vi "Database.Handler.CheckStatus.vi"(8 "error in (no error)":errorcluster, 11 "Data in":T1) -> (0 "error out":errorcluster, 3 "Data out":T1)   [LabVIEW 2016]
uses:
  Database.Global.vi
  Global/ApplicationGlobal.vi
  Tools/EventLog/EventLog.EventSource.ctl
  Tools/Translator/Translator.Message.ctl
  Tools/EventLog/EventLog.New(array).vi
  Database.Handler.Data.Status.ctl
  Database.Handler.Data.Sets.ctl
  Database.Handler.Data.ctl
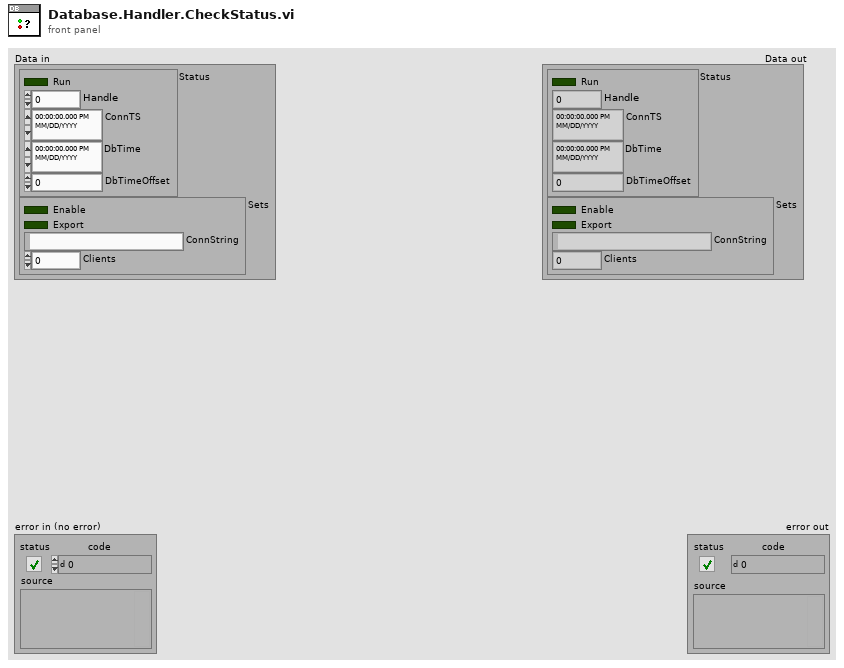
[diagram p1: front panel]
types:
  T1 = typedef "Database.Handler.Data.ctl" = cluster{"Status":T2, "Sets":T3}
  T2 = typedef "Database.Handler.Data.Status.ctl" = cluster{"Run":bool, "Handle":i32, "ConnTS":timestamp, "DbTime":timestamp, "DbTimeOffset":dbl}
  T3 = typedef "Database.Handler.Data.Sets.ctl" = cluster{"Enable":bool, "Export":bool, "ConnString":string, "Clients":i32}
  T4 = typedef "Translator.Message.ctl" = enum16{"-", "Event confirmed", "Log out", "Log in", "Shutdown", "Cancel", "Start", "Continue", "Stop", "On", "Off", "OK", "NOK", "NOK %s", "This", "Prev", "Home", "Work", "In progress...", "Missing", "Empty", "Hardware failure", "Initial", "Error %d >> %s", "Error %d >> %s >> %s", "Starting %s", "Quitting %s", "Configured", "Initializing", "Quitting", "Loading", "Running %s", "Stopped", "Summary", "Do you want to continue?", "Do you want to exit?", "Log out?", "System", "All", "IDLE", "Translating...%s", "Not found", "Alarm %s", "Run", "Skip", "Abort", "Repeat", "Please wait...", "Database disconnected", "Login to database successful", "Login to database failed: %d; %s", "Get process step data for %s", "Changeover off", "Changeover into %s", "Product %s | %s found in cache with status %d at previous station", "Product %s | %s found in database with status %d at previous station", "Product %s | %s not found in cache at previous station", "Product %s | %s not found in database at previous station", "Product %s | %s found in cache with status %d at this station (%d repetion)", "Product %s | %s found in database with status %d at this station (%d repetition)", "Product %s | %s not found in cache at this station", "Product %s | %s not found in database at this station", "Product %s | %s found in cache for component %s | %s", "Product %s | %s found in database for component %s | %s", "Product not found in cache for component %s | %s", "Product not found in database for component %s | %s", "Product %s | %s connected with component %s | %s (cache)", "Product %s | %s connected with component %s | %s (database)", "New data for %s | %s (cache)", "New data for %s | %s (database)", "File %s moved (cache)", "File %s deleted (cache)", "Msg %d >> %s", "PLC LifeBit Failure", "Reconnecting DB", "Reconnecting PLC", "Free disk space is below 1GB - contact technician"}
  T5 = typedef "EventLog.EventSource.ctl" = enum16{"All", "Gui", "Cache", "PLC1", "PLC2", "PLC3", "DB", "DB01", "DB02", "DB03", "DB04", "DB05", "DB06", "DB07", "DB08", "DB09", "DB10", "DB11", "DB12", "DB13", "DB14", "DB15", "DB16"}
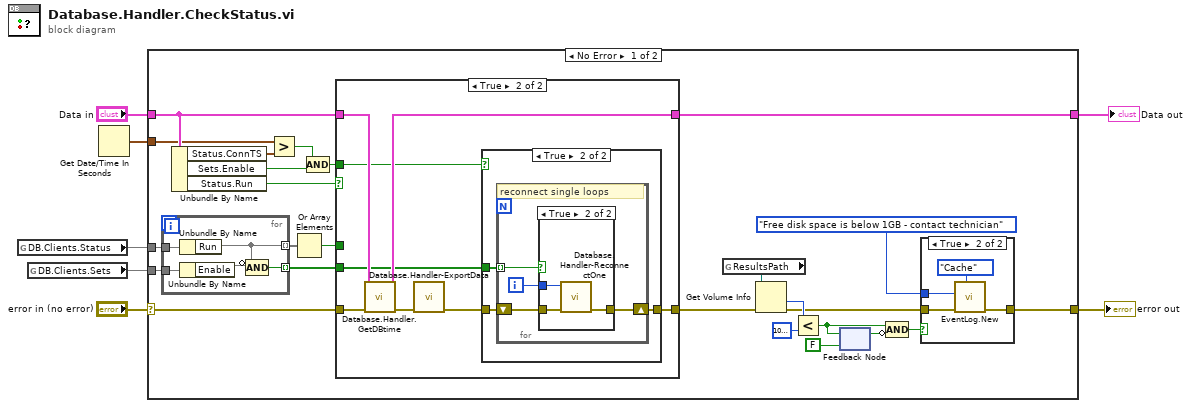
[diagram p0: block diagram]
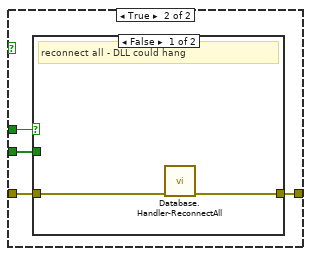
[diagram p4: hidden frame]
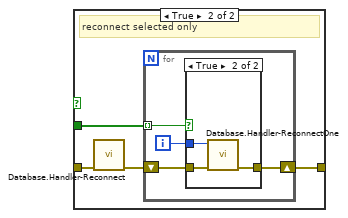
[diagram p5: hidden frame]
diagram:
  n1 = global read "Database.Global.vi" "DB.Clients.Status"() -> (w6)
  n2 = global read "Database.Global.vi" "DB.Clients.Sets"() -> (w5)
  n3 = Get Date/Time In Seconds() -> (seconds since 1Jan1904=w1:timestamp)
  n4 = case shown="No Error" "error in (no error)" {
    selector: "error in (no error)" -> [w29 w89]
    tunnel: "Data in" -> [w28 w88]
    tunnel: w6 -> [w32 _]
    tunnel: w5 -> [w31 _]
    tunnel: [w10 w89] -> w3
    tunnel: [w24 w88] -> w2
    tunnel: w1 -> [w22 _]
    frame No Error {
      n5 = for {
        tunnel: w32 -> [w42]
        tunnel: w31 -> [w41]
        tunnel: [w40] -> w30 mode=indexing
        tunnel: [w38] -> w25 mode=indexing
        n6 = Unbundle By Name(w42) -> ("Run"=w40)
        n7 = Unbundle By Name(w41) -> ("Enable"=w39)
        n8 = Compound Arithmetic op=AND(invert w40, w39) -> (w38:bool)
      }
      n9 = Unbundle By Name(w28) -> ("Status.ConnTS"=w23:timestamp, "Sets.Enable"=w21:bool, "Status.Run"=w27:bool)
      n10 = Greater?(x=w22, y=w23) -> (0:w20:bool)
      n11 = Or Array Elements(Boolean array=w30) -> (logical OR=w26:bool)
      n12 = Compound Arithmetic op=AND(w20, w21) -> (w19:bool)
      n13 = case shown="True" w27 {
        tunnel: w29 -> [w48 w74]
        tunnel: [w47 w70] -> w11
        tunnel: w28 -> [w44 w73]
        tunnel: w26 -> [w46 _]
        tunnel: w25 -> [w45 w69]
        tunnel: [w44 w72] -> w24
        tunnel: w19 -> [w43 w68]
        frame False {
          n14 = case shown="False" w43 {
            tunnel: w48 -> [w49 w52]
            tunnel: [w49 w51] -> w47
            tunnel: w46 -> [_ w53]
            tunnel: w45 -> [_ w50]
            frame False {
            }
            frame True {
              n15 = case shown="False" w53 {
                tunnel: w52 -> [w55 w57]
                tunnel: [w54 w59] -> w51
                tunnel: w50 -> [_ w58]
                frame False {
                  # "reconnect all - DLL could hang"
                  n16 = call "Database.Handler-ReconnectAll.vi"("error in"=w55) -> ("error out"=w54:errorcluster)  [unwired: 10 in]
                }
                frame True {
                  # "reconnect selected only"
                  n17 = call "Database.Handler-Reconnect.vi"("error in"=w57) -> ("error out"=w56:errorcluster)  [unwired: 10 in]
                  n18 = for {
                    shift-right: [w60] -> w59
                    shift-left: w56 -> [w63]
                    tunnel: w58 -> [w61] mode=indexing
                    i -> [w62]
                    n19 = case shown="True" w61 {
                      tunnel: w63 -> [w64 w67]
                      tunnel: w62 -> [_ w65]
                      tunnel: [w64 w66] -> w60
                      frame False {
                      }
                      frame True {
                        n20 = call "Database.Handler-ReconnectOne.vi"("error in"=w67, "ClientIdx"=w65) -> ("error out"=w66:errorcluster)  [unwired: 9 in]
                      }
                    }
                  }
                }
              }
            }
          }
        }
        frame True {
          n21 = call "Database.Handler.GetDBtime.vi"("error in (no error)"=w74, "Data in"=w73) -> ("error out"=w75:errorcluster, "Data out"=w72:T1)  [unwired: 8 in]
          n22 = call "Database.Handler-ExportData.vi"("error in"=w75) -> ("error out"=w71:errorcluster)  [unwired: 10 in]
          n23 = case shown="True" w68 {
            tunnel: w71 -> [w76 w79]
            tunnel: [w76 w78] -> w70
            tunnel: w69 -> [_ w77]
            frame False {
            }
            frame True {
              n24 = for {
                shift-right: [w80] -> w78
                shift-left: w79 -> [w83]
                tunnel: w77 -> [w81] mode=indexing
                i -> [w82]
                # "reconnect single loops"
                n25 = case shown="True" w81 {
                  tunnel: w83 -> [w84 w87]
                  tunnel: w82 -> [_ w85]
                  tunnel: [w84 w86] -> w80
                  frame False {
                  }
                  frame True {
                    n26 = call "Database.Handler-ReconnectOne.vi"("error in"=w87, "ClientIdx"=w85) -> ("error out"=w86:errorcluster)  [unwired: 9 in]
                  }
                }
              }
            }
          }
        }
      }
      n27 = global read "ApplicationGlobal.vi" "ResultsPath"() -> (w18:path)
      n28 = Get Volume Info(8:w11, 11:w18) -> (0:w12:errorcluster, 1:w17:i64)  [unwired: 4 out]
      n29 = Less?(x=w17, y=i64 1000000000) -> (x < y?=w15:bool)
      n30 = feedback #1(FALSE) -> (w13:bool)
      n31 = feedback-in #1(w15) -> ()
      n32 = Compound Arithmetic op=AND(w15, invert w13) -> (w9:bool)
      n33 = case shown="True" w9 {
        tunnel: w12 -> [w33 w37]
        tunnel: Translator.Message."Free disk space is below 1GB - contact technician" ("msg") -> [_ w35]
        tunnel: [w33 w34] -> w10
        frame False {
        }
        frame True {
          n34 = call-poly "EventLog.New.vi"("Source (All)"=EventLog.EventSource."Cache", "error in (no error)"=w37, "Message (-)"=w35) -> ("error out"=w34:errorcluster)  [unwired: 7 in, 1 out]
        }
      }
    }
    frame Error {
    }
  }
  "Data out" <- w2
  "error out" <- w3
